vi "Validate Limit.vi"(5 "GU Pass Count Disp":refnum<vi>, 7 "Info Disp":refnum<vi>, 8 "error in":errorcluster, 9 "Min Pass Num Per Batch":i32, 10 "Limit Status":T1, 11 "IsCalibration":bool) -> (0 "error out":errorcluster, 3 "Update Offset":bool)   [LabVIEW 2020, in "GUCalibration2.lvlib"]
uses:
  GUCalibration2.lvlib
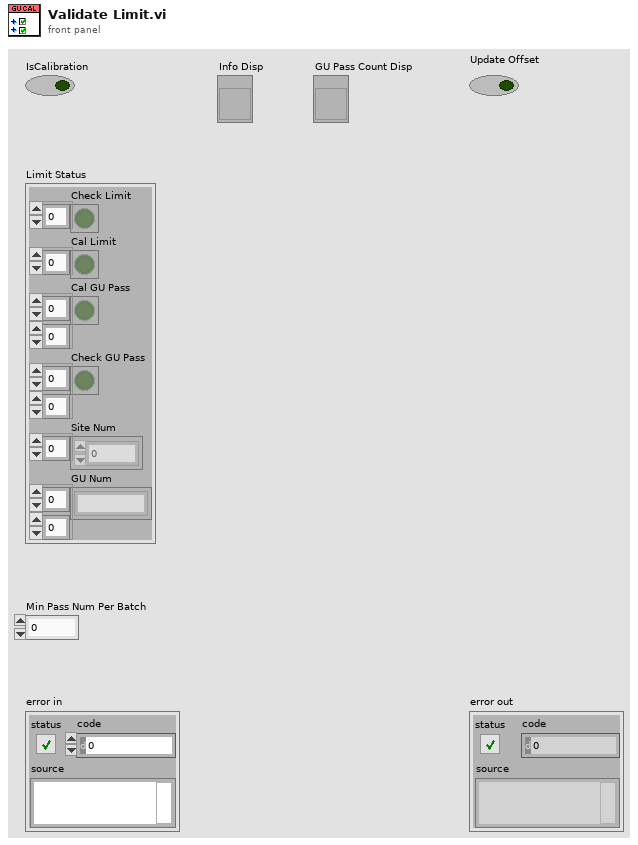
[diagram p1: front panel]
types:
  T1 = cluster{"Check Limit":bool[], "Cal Limit":bool[], "Cal GU Pass":bool[][], "Check GU Pass":bool[][], "Site Num":i32[], "GU Num":string[][]}
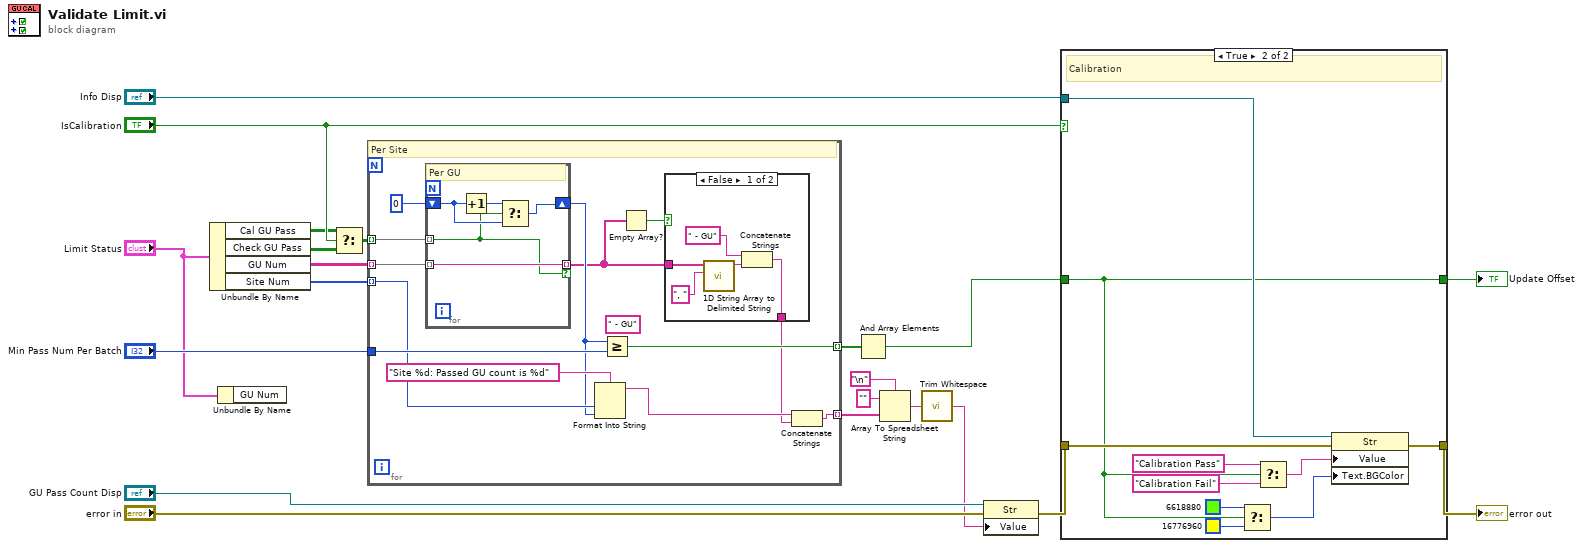
[diagram p0: block diagram]
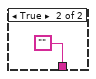
[diagram p2: hidden frame]
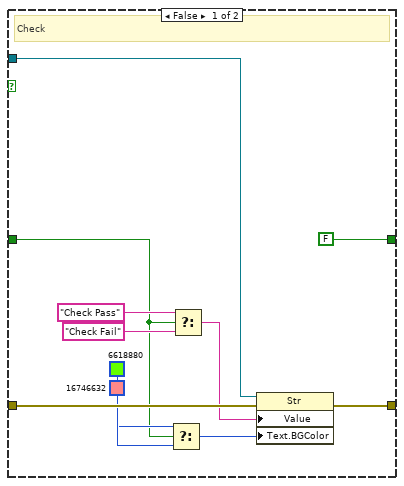
[diagram p3: hidden frame]
diagram:
  n1 = Unbundle By Name("Limit Status") -> ("Cal GU Pass"=w14:bool[][], "Check GU Pass"=w13:bool[][], "GU Num"=w1:string[][], "Site Num"=w11:i32[])
  n2 = Unbundle By Name("Limit Status") -> ()  [unwired: 1 out]
  n3 = Select(t=w14, s="IsCalibration", f=w13) -> (s? t:f=w15:bool[][])
  n4 = for {
    tunnel: w15 -> [w34] mode=indexing
    tunnel: "Min Pass Num Per Batch" -> [w32]
    tunnel: [w31] -> w17 mode=indexing
    tunnel: w11 -> [w29] mode=indexing
    tunnel: [w23] -> w7 mode=indexing
    tunnel: w1 -> [w26] mode=indexing
    (unwired) " - GU"
    # "Per Site"
    n5 = for {
      tunnel: w34 -> [w41] mode=indexing
      shift-right: [w44] -> w27
      shift-left: 0 -> [w43]
      tunnel: w26 -> [w42] mode=indexing
      tunnel: [w42] -> w24 mode=indexing if=w41
      # "Per GU"
      n6 = Increment(x=w43) -> (x+1=w45:i32)
      n7 = Select(t=w45, s=w41, f=w43) -> (s? t:f=w44:i32)
    }
    n8 = Format Into String(format string="Site %d: Passed GU count is %d", w29, w27) -> (resulting string=w28:string)  [unwired: 2 in, 1 out]
    n9 = Greater Or Equal?(x=w27, y=w32) -> (x >= y?=w31:bool)
    n10 = Empty Array?(array=w24) -> (empty?=w25:bool)
    n11 = case shown="False" w25 {
      tunnel: w24 -> [w38 _]
      tunnel: [w35 ""] -> w22
      frame False {
        n12 = call <vilib>:"1D String Array to Delimited String.vi"("delimiter"=", ", "string array"=w38) -> ("delimited string"=w37:string)  [unwired: 9 in]
        n13 = Concatenate Strings(" - GU" ("string"), w37) -> (w35:string)
      }
      frame True {
      }
    }
    n14 = Concatenate Strings(w28, w22) -> (w23:string)
  }
  n15 = And Array Elements(Boolean array=w17) -> (logical AND=w12:bool)
  n16 = Array To Spreadsheet String(delimiter (Tab)="\n", array=w7, 3:"" ("format string")) -> (spreadsheet string=w4:string)
  n17 = call <vilib>:"Trim Whitespace.vi"("string"=w4) -> ("trimmed string"=w3:string)  [unwired: 1 in]
  n18 = property class="Str"(reference="GU Pass Count Disp", error in="error in", "Value"=w3) -> (error out=w8:errorcluster)  [unwired: 1 out]
  n19 = case shown="True" "IsCalibration" {
    tunnel: w12 -> [w46 w58]
    tunnel: [FALSE w58] -> w21
    tunnel: "Info Disp" -> [w51 w64]
    tunnel: w8 -> [w53 w66]
    tunnel: [w52 w65] -> w20
    frame False {
      # "Check"
      n20 = Select(t=u32 6618880, s=w46, f=u32 16746632) -> (s? t:f=w47:u32)
      n21 = Select(t="Check Pass", s=w46, f="Check Fail") -> (s? t:f=w50:string)
      n22 = property class="Str"(reference=w51, error in=w53, "Value"=w50, "Text.BGColor"=w47) -> (error out=w52:errorcluster)  [unwired: 1 out]
    }
    frame True {
      # "Calibration"
      n23 = Select(t=u32 6618880, s=w58, f=u32 16776960) -> (s? t:f=w61:u32)
      n24 = Select(t="Calibration Pass", s=w58, f="Calibration Fail") -> (s? t:f=w59:string)
      n25 = property class="Str"(reference=w64, error in=w66, "Value"=w59, "Text.BGColor"=w61) -> (error out=w65:errorcluster)  [unwired: 1 out]
    }
  }
  "error out" <- w20
  "Update Offset" <- w21
